vi "Gas_Density.vi"(1 "Pressure (mbars)":dbl=1000.0 format="%.2f", 2 "Temperature (deg C)":dbl format="%.2f", 3 "Gas Name":string) -> (0 "Density Kg/m3":dbl=nan format="%.4f")   [LabVIEW 2016]
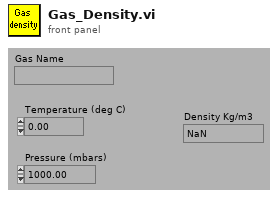
[diagram p1: front panel]
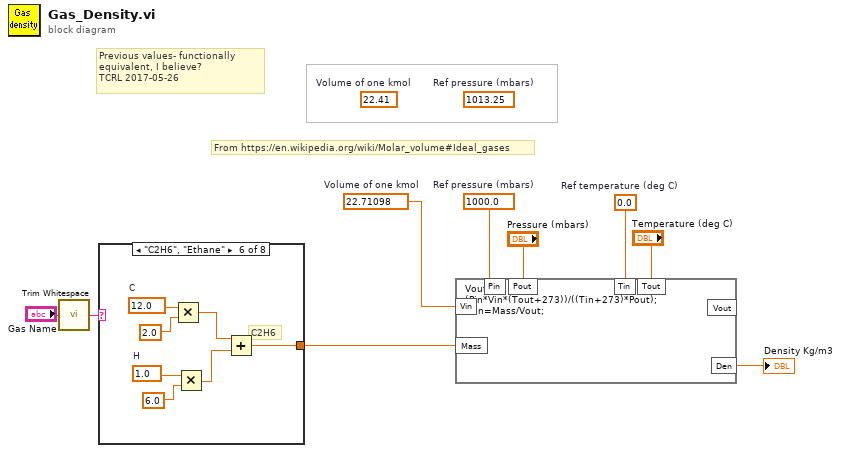
[diagram p0: block diagram]
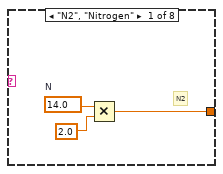
[diagram p2: hidden frame]
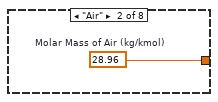
[diagram p3: hidden frame]
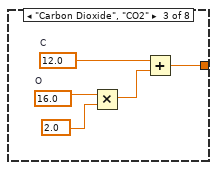
[diagram p4: hidden frame]
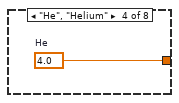
[diagram p5: hidden frame]
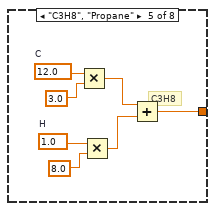
[diagram p6: hidden frame]
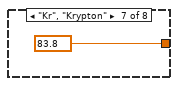
[diagram p7: hidden frame]
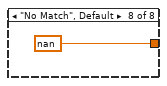
[diagram p8: hidden frame]
diagram:
  (unwired) 1013.25  # Ref pressure (mbars)
  (unwired) 22.41  # Volume of one kmol
  w7 = 1000.0  # Ref pressure (mbars)
  w6 = 0.0  # Ref temperature (deg C)
  w9 = 22.71098  # Volume of one kmol
  # "Previous values- functionally equivalent, I believe?\nTCRL 2017-05-26"
  # "From https://en.wikipedia.org/wiki/Molar_volume#Ideal_gases"
  n1 = call <vilib>:"Trim Whitespace.vi"("string"="Gas Name") -> ("trimmed string"=w1:string)  [unwired: 1 in]
  n2 = case shown="\"C2H6\", \"Ethane\"" w1 {
    tunnel: [w10 w13 w14 w19 w20 w27 83.8 nan] -> w8
    frame "N2", "Nitrogen" {
      w12 = 14.0  # N
      # "N2"
      n3 = Multiply(x=w12, y=2.0) -> (x*y=w10:dbl)
    }
    frame "Air" {
      w13 = 28.96  # Molar Mass of Air (kg/kmol)
    }
    frame "Carbon Dioxide", "CO2" {
      w18 = 12.0  # C
      w15 = 16.0  # O
      n4 = Multiply(x=w15, y=2.0 ("O")) -> (x*y=w17:dbl)
      n5 = Add(x=w18, y=w17) -> (x+y=w14:dbl)
    }
    frame "He", "Helium" {
      w19 = 4.0  # He
    }
    frame "C3H8", "Propane" {
      w24 = 1.0  # H
      w25 = 12.0  # C
      # "C3H8"
      n6 = Multiply(x=w25, y=3.0) -> (x*y=w22:dbl)
      n7 = Multiply(x=w24, y=8.0) -> (x*y=w21:dbl)
      n8 = Add(x=w22, y=w21) -> (x+y=w20:dbl)
    }
    frame "C2H6", "Ethane" {
      w31 = 1.0  # H
      w32 = 12.0  # C
      # "C2H6"
      n9 = Multiply(x=w32, y=2.0) -> (x*y=w29:dbl)
      n10 = Multiply(x=w31, y=6.0) -> (x*y=w28:dbl)
      n11 = Add(x=w29, y=w28) -> (x+y=w27:dbl)
    }
    frame "Kr", "Krypton" {
    }
    frame "No Match", Default {
    }
  }
  n12 = formula code="Vout=\n(Pin*Vin*(Tout+273))/((Tin+273)*Pout);\nDen=Mass/Vout;"("Pin"=w7, "Vin"=w9, "Tout"="Temperature (deg C)", "Tin"=w6, "Pout"="Pressure (mbars)", "Mass"=w8) -> ("Den"=→"Density Kg/m3":dbl)  [unwired: 1 out]
